vi "Daten kopieren auf PC.vi"(8 "error in":errorcluster, 10 "Pfad Communication":path, 11 "Pfad PC":path caption="Lokaler Pfad") -> (0 "error out":errorcluster, 2 "ohne Fehler":bool)   [LabVIEW 2020, in "Backup.lvlib"]
uses:
  Backup.lvlib
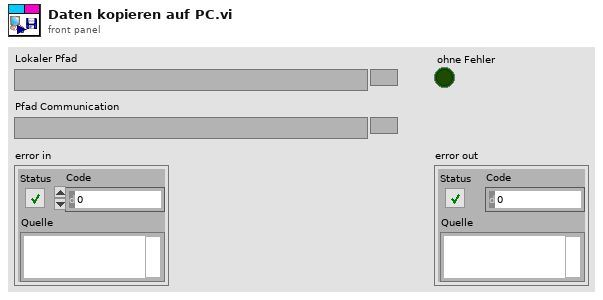
[diagram p1: front panel]
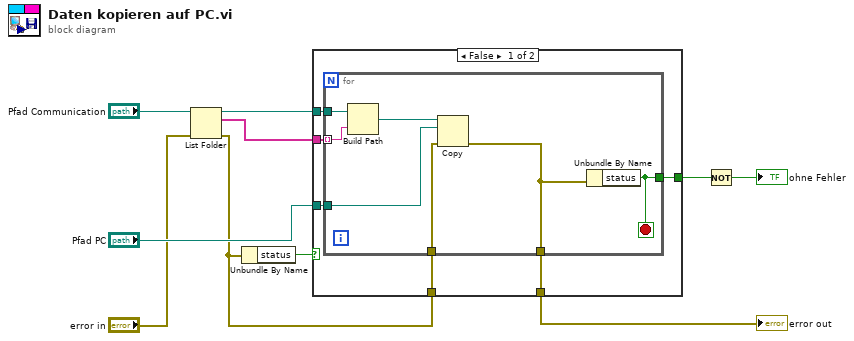
[diagram p0: block diagram]
diagram:
  n1 = List Folder(path="Pfad Communication", error in="error in") -> (path out=w1:path, filenames=w3:string[], error out=w4:errorcluster)  [unwired: 2 in, 1 out]
  n2 = Unbundle By Name(w4) -> ("status"=w8:bool)
  n3 = case shown="False" w8 {
    selector: w8 -> [_ w25]
    tunnel: "Pfad PC" -> [w16 _]
    tunnel: w4 -> [w15 w24]
    tunnel: [w13 w25] -> w7
    tunnel: [w14 w24] -> w6
    tunnel: w3 -> [w12 _]
    tunnel: w1 -> [w11 _]
    frame False {
      n4 = for {
        tunnel: w16 -> [w23]
        tunnel: w15 -> [w22]
        tunnel: [w21] -> w14
        tunnel: [w20] -> w13
        tunnel: w12 -> [w19] mode=indexing
        tunnel: w11 -> [w18]
        stop <- w20 stop-if-true
        n5 = Build Path(base path=w18, name or relative path=w19) -> (appended path=w17:path)
        n6 = Copy(8:w22, 10:w23, 11:w17) -> (0:w21:errorcluster)  [unwired: 2 in, 2 out]
        n7 = Unbundle By Name(w21) -> ("status"=w20:bool)
      }
    }
    frame True {
    }
  }
  "error out" <- w6
  n8 = Not(x=w7) -> (.not. x?=→"ohne Fehler":bool)
